vi "2D force plotting.vi"(5 "Trap positions":cluster{"X":dbl[], "Y":dbl[]}[](array[cluster]), 6 "Calibration":u16(ring)=2 items=["None", "Position", "Force"], 7 "Bead sizes":dbl[](array[numeric]), 8 "Raw Data":waveform(dbl)[](array[waveform]), 9 "Deflections":waveform(dbl)[](array[waveform]), 10 "Forces":waveform(dbl)[](array[waveform]), 11 "Absolute Positions":waveform(dbl)[](array[waveform])) -> (0 "Output waveforms":waveform(dbl)[](array[waveform]), 1 "Output":T1={"A_X"=0.0605018, "A_Y"=0.0, "B_X"=0.0507675, "B_Y"=0.0, "C_X"=0.0, "C_Y"=0.0}, 2 "Junctions":cluster{"X":dbl[], "Y":dbl[]}[](array[cluster]), 3 "deflection lines":cluster{"X":dbl[], "Y":dbl[]}[](array[cluster]), 4 "tether sizes":dbl[][](array[numeric]))   [LabVIEW 2014]
uses:
  <vilib>/Analysis/baseanly.llb/Mean (DBL).vi
  <vilib>/imath/engines/lvmath2/RunTimeEngine/IndexRead/NIMS M(S,$).vi
  <instcachedir>/0/NIMS M(S,$)_F24F360562DE41D8BE234322A2E15C65.lvgen/NIMS M(S,$)_F24F360562DE41D8BE234322A2E15C65_000.vi
  <vilib>/imathl/engines/lvmath/Functions/Error Handling/Create Error.vi
  <vilib>/imath/engines/lvmath2/RunTimeEngine/ArithmeticOperatorToken/NIMS_ArithmeticOperator_minus.vi
  <instcachedir>/0/NIMS_ArithmeticOperator_minus_39C0593E74DA4138ACA2AB742906488D.lvgen/NIMS_ArithmeticOperator_minus_39C0593E74DA4138ACA2AB742906488D_003.vi
  <vilib>/imath/engines/lvmath2/RunTimeEngine/ArithmeticOperatorToken/NIMS_ArithmeticOperator_times.vi
  <instcachedir>/0/NIMS_ArithmeticOperator_times_2EFF5B13FCA4492A81D59089AD809F54.lvgen/NIMS_ArithmeticOperator_times_2EFF5B13FCA4492A81D59089AD809F54_000.vi
  <vilib>/imath/engines/lvmath2/RunTimeEngine/ArithmeticOperatorToken/NIMS_ArithmeticOperator_rightdiv.vi
  <instcachedir>/0/NIMS_ArithmeticOperator_rightdiv_1C32D12ACC084D698DD85086C55578F5.lvgen/NIMS_ArithmeticOperator_rightdiv_1C32D12ACC084D698DD85086C55578F5_000.vi
  <vilib>/imath/engines/lvmath2/RunTimeEngine/ErrorHandling/NIMS_Create Error From Enums.vi
  <vilib>/imath/engines/lvmath2/RunTimeEngine/BuiltInFunctions/length/NIMS_length(GV).vi
  <instcachedir>/0/NIMS_length(GV)_08A3D13377FD4E4B96F5795FBF3698FA.lvgen/NIMS_length(GV)_08A3D13377FD4E4B96F5795FBF3698FA_000.vi
  <vilib>/imath/engines/lvmath2/RunTimeEngine/BuiltInFunctions/zeros/NIMS_M=zeros(I32,I32).vi
  <vilib>/imath/engines/lvmath2/RunTimeEngine/BuiltInFunctions/zeros/NIMS_V=zeros(I32,I32).vi
  <vilib>/imath/engines/lvmath2/RunTimeEngine/ArithmeticOperatorToken/NIMS_ArithmeticOperator_plus.vi
  <instcachedir>/0/NIMS_ArithmeticOperator_plus_48D6EAACA5D645B09F7EC9C016C2DEA8.lvgen/NIMS_ArithmeticOperator_plus_48D6EAACA5D645B09F7EC9C016C2DEA8_004.vi
  <vilib>/imath/engines/lvmath2/RunTimeEngine/IndexReplace/NIMS M(S,$)=V.vi
  <instcachedir>/0/NIMS M(S,$)=V_8321FD9A786642FB877A2933E8B48D2A.lvgen/NIMS M(S,$)=V_8321FD9A786642FB877A2933E8B48D2A_000.vi
  <vilib>/imath/engines/lvmath2/RunTimeEngine/BuiltInFunctions/mean/NIMS_RRow=mean(RM,I32).vi
  <vilib>/imath/engines/lvmath2/RunTimeEngine/IndexRead/NIMS V(S).vi
  <instcachedir>/0/NIMS V(S)_0488751826AF41519A22953C041130DC.lvgen/NIMS V(S)_0488751826AF41519A22953C041130DC_000.vi
  <instcachedir>/0/NIMS M(S,$)=V_8321FD9A786642FB877A2933E8B48D2A.lvgen/NIMS M(S,$)=V_8321FD9A786642FB877A2933E8B48D2A_001.vi
  <vilib>/imath/engines/lvmath2/RunTimeEngine/NodeEndStatement/NIMS_NodeEndStatement_Output.vi
  <instcachedir>/0/NIMS_NodeEndStatement_Output_53EC0D466D134D7ABD903AC30B43404B.lvgen/NIMS_NodeEndStatement_Output_53EC0D466D134D7ABD903AC30B43404B_003.vi
  <instcachedir>/0/NIMS_NodeEndStatement_Output_53EC0D466D134D7ABD903AC30B43404B.lvgen/NIMS_NodeEndStatement_Output_53EC0D466D134D7ABD903AC30B43404B_005.vi
  <instcachedir>/0/NIMS_NodeEndStatement_Output_53EC0D466D134D7ABD903AC30B43404B.lvgen/NIMS_NodeEndStatement_Output_53EC0D466D134D7ABD903AC30B43404B_002.vi
  <vilib>/imath/engines/lvmath2/RunTimeEngine/ErrorHandling/NIMS_Finalize Error.vi
  <vilib>/Analysis/NI_AALBase.lvlib
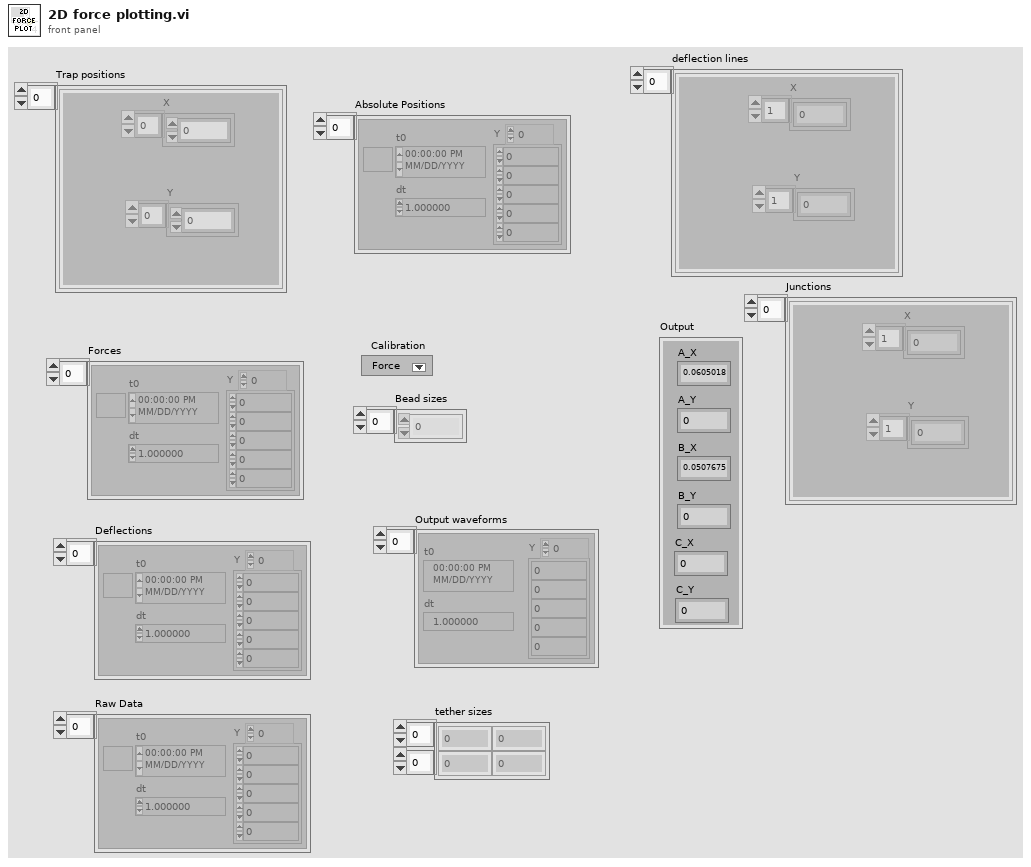
[diagram p1: front panel]
types:
  T1 = cluster{"A_X":dbl, "A_Y":dbl, "B_X":dbl, "B_Y":dbl, "C_X":dbl, "C_Y":dbl}
  T2 = cluster{"[0]":dbl, "[1]":dbl, "[2]":dbl, "[3]":dbl, "[4]":dbl, "[5]":dbl}
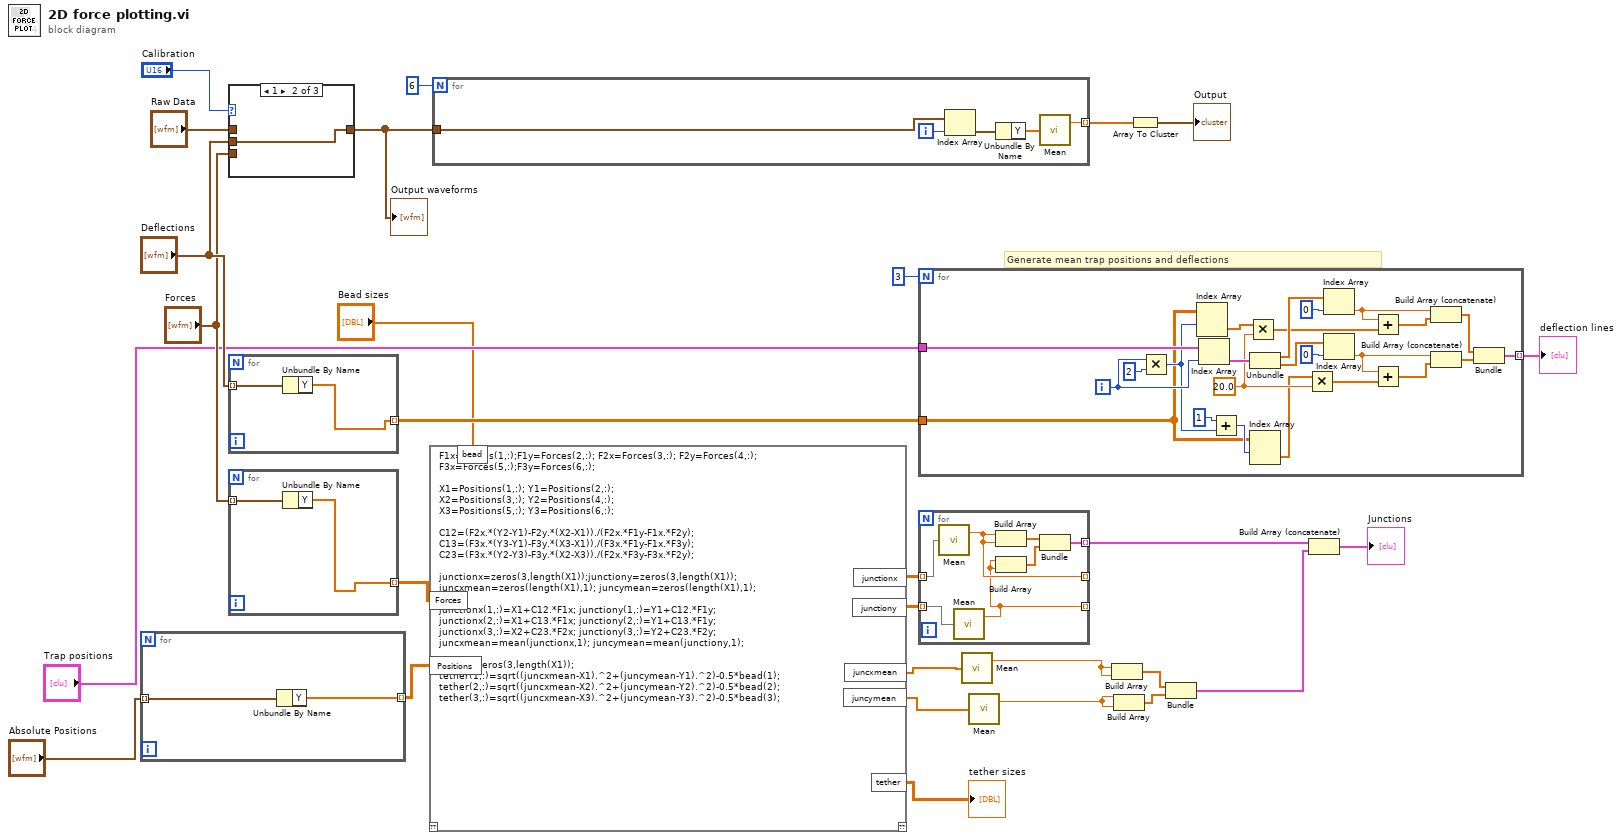
[diagram p0: block diagram]
diagram:
  # "Generate mean trap positions and deflections"
  n1 = for {
    tunnel: "Absolute Positions" -> [w30] mode=indexing
    tunnel: [w29] -> w6 mode=indexing
    n2 = Unbundle By Name(w30) -> ("Y"=w29:dbl[])
  }
  n3 = case shown="1" "Calibration" {
    tunnel: "Forces" -> [_ _ w33]
    tunnel: [w31 w32 w33] -> w26
    tunnel: "Deflections" -> [_ w32 _]
    tunnel: "Raw Data" -> [w31 _ _]
    frame 0, Default {
    }
    frame 1 {
    }
    frame 2 {
    }
  }
  "Output waveforms" <- w26
  n4 = for {
    tunnel: "Deflections" -> [w35] mode=indexing
    tunnel: [w34] -> w16 mode=indexing
    n5 = Unbundle By Name(w35) -> ("Y"=w34:dbl[])
  }
  n6 = for {
    tunnel: "Forces" -> [w37] mode=indexing
    tunnel: [w36] -> w18 mode=indexing
    n7 = Unbundle By Name(w37) -> ("Y"=w36:dbl[])
  }
  n8 = mathscript code="F1x=Forces(1,:);F1y=Forces(2,:); F2x=Forces(3,:); F2y=Forces(4,:);\nF3x=Forces(5,:);F3y=Forces(6,:);\n\nX1=Positions(1,:); Y1=Positions(2,:); \nX2=Positions(3,:); Y2=Positions(4,:);\nX3=Positions(5,:); Y3=Positions(6,:);\n\nC12=(F2x.*(Y2-Y1)-F2y.*(X2-X1))./(F2x.*F1y-F1x.*F2y);\nC13=(F3x.*(Y3-Y1)-F3y.*(X3-X1))./(F3x.*F1y-F1x.*F3y);\nC23=(F3x.*(Y2-Y3)-F3y.*(X2-X3))./(F2x.*F3y-F3x.*F2y);\n\njunctionx=zeros(3,length(X1));junctiony=zeros(3,length(X1));\njuncxmean=zeros(length(X1),1); juncymean=zeros(length(X1),1);\n\njunctionx(1,:)=X1+C12.*F1x; junctiony(1,:)=Y1+C12.*F1y;\njunctionx(2,:)=X1+C13.*F1x; junctiony(2,:)=Y1+C13.*F1y;\njunctionx(3,:)=X2+C23.*F2x; junctiony(3,:)=Y2+C23.*F2y;\njuncxmean=mean(junctionx,1); juncymean=mean(junctiony,1);\n\ntether=zeros(3,length(X1));\ntether(1,:)=sqrt((juncxmean-X1).^2+(juncymean-Y1).^2)-0.5*bead(1);\ntether(2,:)=sqrt((juncxmean-X2).^2+(juncymean-Y2).^2)-0.5*bead(2);\ntether(3,:)=sqrt((juncxmean-X3).^2+(juncymean-Y3).^2)-0.5*bead(3);"("Forces"=w18, "Positions"=w6, "bead"="Bead sizes") -> ("junctionx"=w15:dbl[][], "junctiony"=w14:dbl[][], "juncxmean"=w5:dbl[], "juncymean"=w3:dbl[], "tether"=→"tether sizes":cdb[][])  [unwired: 1 in, 1 out]
  n9 = for {
    N: 6 -> [_]
    tunnel: w26 -> [w41]
    tunnel: [w38] -> w24 mode=indexing
    i -> [w42]
    n10 = Index Array(array=w41, index=w42) -> (element=w40:waveform(dbl))
    n11 = Unbundle By Name(w40) -> ("Y"=w39:dbl[])
    n12 = call-poly <vilib>:"Mean.vi"("X"=w39) -> ("mean"=w38:dbl)  [unwired: 1 out]
  }
  n13 = for {
    N: 3 -> [_]
    tunnel: "Trap positions" -> [w66]
    tunnel: [w55] -> w21 mode=indexing
    tunnel: w16 -> [w44]
    i -> [w64]
    w47 = 20.0
    n14 = Multiply(x=w64, y=2) -> (x*y=w60:i32)
    n15 = Index Array(array=w44, index (row)=w60) -> (element=w45:dbl[])  [unwired: 1 in]
    n16 = Index Array(array=w66, index=w64) -> (element=w65:cluster{"X":dbl[], "Y":dbl[]})
    n17 = Add(x=1, y=w60) -> (x+y=w61:i32)
    n18 = Multiply(x=w45, y=w47) -> (x*y=w46:dbl[])
    n19 = Unbundle(w65) -> ("X"=w54:dbl[], "Y"=w53:dbl[])
    n20 = Index Array(array=w44, index (row)=w61) -> (element=w43:dbl[])  [unwired: 1 in]
    n21 = Multiply(x=w43, y=w47) -> (x*y=w48:dbl[])
    n22 = Index Array(array=w54, index=0) -> (element=w50:dbl)
    n23 = Index Array(array=w53, index=0) -> (element=w49:dbl)
    n24 = Add(x=w50, y=w46) -> (x+y=w57:dbl[])
    n25 = Add(x=w49, y=w48) -> (x+y=w56:dbl[])
    n26 = Build Array (concatenate)(w50, w57) -> (w59:dbl[])
    n27 = Build Array (concatenate)(w49, w56) -> (w58:dbl[])
    n28 = Bundle(w59, w58) -> (w55:cluster{dbl[], dbl[]})  [unwired: 1 in]
  }
  "deflection lines" <- w21
  n29 = for {
    tunnel: w15 -> [w70] mode=indexing
    tunnel: w14 -> [w68] mode=indexing
    tunnel: [w71] -> w13 mode=indexing
    tunnel: [w69] -> _ mode=indexing
    tunnel: [w67] -> _ mode=indexing
    n30 = call-poly <vilib>:"Mean.vi"("X"=w70) -> ("mean"=w69:dbl)  [unwired: 1 out]
    n31 = call-poly <vilib>:"Mean.vi"("X"=w68) -> ("mean"=w67:dbl)  [unwired: 1 out]
    n32 = Build Array(w69, w69) -> (w73:dbl[])
    n33 = Build Array(w67, w67) -> (w72:dbl[])
    n34 = Bundle(w73, w72) -> (w71:cluster{dbl[], dbl[]})  [unwired: 1 in]
  }
  n35 = call-poly <vilib>:"Mean.vi"("X"=w5) -> ("mean"=w4:dbl)  [unwired: 1 out]
  n36 = call-poly <vilib>:"Mean.vi"("X"=w3) -> ("mean"=w2:dbl)  [unwired: 1 out]
  n37 = Build Array(w4, w4) -> (w11:dbl[])
  n38 = Build Array(w2, w2) -> (w10:dbl[])
  n39 = Array To Cluster(array=w24) -> (cluster=→"Output":T2)
  n40 = Bundle(w11, w10) -> (w9:cluster{dbl[], dbl[]})  [unwired: 1 in]
  n41 = Build Array (concatenate)(w13, w9) -> (→"Junctions":cluster{dbl[], dbl[]}[])
